vi "Jc.vi"() -> ()   [LabVIEW 2020]
panel:
  out "Jc sphere divided":dbl=0.002401644001219178 format="%#_e A/cm^2"
  out "Jc disk divided":dbl=51.642493776215986 format="%#_e A/cm^2"
  out "Jc sphere":dbl=0.002401644001219178 format="%#_e A/cm^2"
  out "Magnetization sphere":dbl=88.94276648750413 format="%#_g emu/cm^3"
  in  "thickness":dbl=0.00028 format="%#_6f cm"
  out "V disc":dbl=1.588860484553038e-08 format="%#_g cm^3"
  out "Jc disk":dbl=0.06432975003265656 format="%#_e A/cm^2"
  out "Magnetization disk":dbl=1800.032178913774 format="%#_g emu/cm^3"
  in  "Moment":dbl=2.86e-05 format="%#_6e emu"
  out "V sphere":dbl=3.2155509806430535e-07 format="%#_g cm^3"
  in  "R":dbl=0.00425 format="%#_6f cm"
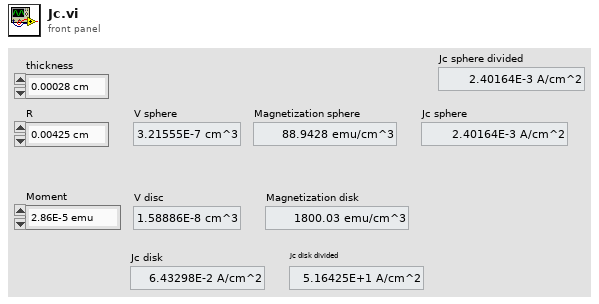
[diagram p1: front panel]
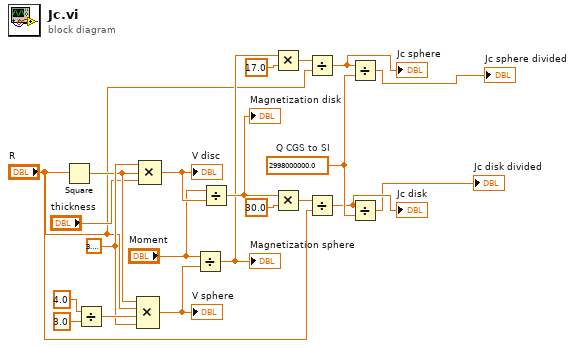
[diagram p0: block diagram]
diagram:
  w7 = 2998000000.0  # Q CGS to SI
  w16 = 3.141592653589793
  n1 = Square(x="R") -> (x^2=w15:dbl)
  n2 = Divide(x=4.0, y=3.0) -> (x/y=w19:dbl)
  n3 = Compound Arithmetic op=MULTIPLY(w15, "R", w19, w16) -> (w11:dbl)
  "V sphere" <- w11
  n4 = Compound Arithmetic op=MULTIPLY(w16, w15, "thickness") -> (w14:dbl)
  "V disc" <- w14
  n5 = Divide(x="Moment", y=w11) -> (x/y=w2:dbl)
  "Magnetization sphere" <- w2
  n6 = Divide(x="Moment", y=w14) -> (x/y=w10:dbl)
  "Magnetization disk" <- w10
  n7 = Multiply(x=w2, y=17.0) -> (x*y=w8:dbl)
  n8 = Multiply(x=w10, y=30.0) -> (x*y=w17:dbl)
  n9 = Divide(x=w8, y="R") -> (x/y=w5:dbl)
  "Jc sphere" <- w5
  n10 = Divide(x=w17, y="R") -> (x/y=w6:dbl)
  "Jc disk" <- w6
  n11 = Divide(x=w5, y=w7) -> (x/y=→"Jc sphere divided":dbl)
  n12 = Divide(x=w6, y=w7) -> (x/y=→"Jc disk divided":dbl)
